vi "Configure HSDIO.vi"(8 "error in (no error)":errorcluster, 11 "HDSIO_Settings":T3={"HSDIO VISA"="6556_0", "Waveform Directory"=path "C:/Users/user/Documents/AD2240/Waveforms/RFFE6", "logic family "=8, "Clock Rate"=20000000.0, "channel list (Clock,Data)"="2,0,6"} {"Clock Rate" format="%.2p"; "logic family" items=["5.0V Logic"=5, "3.3V Logic"=6, "2.5V Logic"=7, "1.8V Logic"=8, "1.5V Logic"=80, "1.2V Logic"=81]}) -> (0 "error out":errorcluster, 3 "HSDIO Sessions":T1)   [LabVIEW 2013]
uses:
  <instrlib>/niHSDIO/niHSDIO.llb/niHSDIO_ctl Voltage Logic Family Values (Ring).ctl
  <instrlib>/niHSDIO/niHSDIO.llb/niHSDIO_ctl Trigger Script - trigID Values (Ring).ctl
  <instrlib>/niHSDIO/niHSDIO.llb/niHSDIO_ctl Generation Mode Values (Ring).ctl
  <instrlib>/niHSDIO/niHSDIO.llb/niHSDIO_ctl Data Position Values (Ring).ctl
  <instrlib>/niHSDIO/niHSDIO.llb/niHSDIO_ctl Trigger Source Values (Ring).ctl
  <instrlib>/niHSDIO/niHSDIO.llb/niHSDIO_ctl Exported Signal Name Values (Ring).ctl
  <instrlib>/niHSDIO/niHSDIO.llb/niHSDIO Configure Data Voltage Logic Family.vi
  <instrlib>/niHSDIO/niHSDIO.llb/niHSDIO Configure Initial State (String).vi
  <instrlib>/niHSDIO/niHSDIO.llb/niHSDIO Configure Idle State (String).vi
  <instrlib>/niHSDIO/niHSDIO.llb/niHSDIO Configure Software Script Trigger.vi
  <instrlib>/niHSDIO/niHSDIO.llb/niHSDIO Configure Digital Edge Start Trigger.vi
  <instrlib>/niHSDIO/niHSDIO.llb/niHSDIO Write Named Waveform From File (HWS).vi
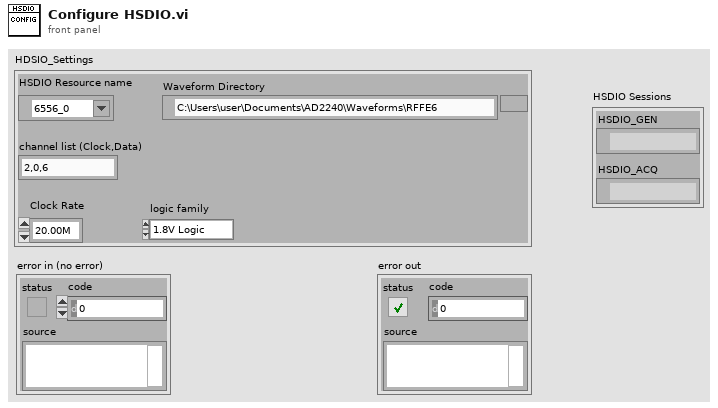
[diagram p1: front panel]
types:
  T1 = cluster{"HSDIO_ACQ":refnum<k15>, "HSDIO_GEN":refnum<k15>}
  T2 = typedef "niHSDIO_ctl Voltage Logic Family Values (Ring).ctl" = i32
  T3 = cluster{"HSDIO VISA":refnum<k15>, "Waveform Directory":path, "logic family ":T2, "Clock Rate":dbl, "channel list (Clock,Data)":string}
  T4 = typedef "niHSDIO_ctl Exported Signal Name Values (Ring).ctl" = u16
  T5 = typedef "niHSDIO_ctl Trigger Source Values (Ring).ctl" = string
  T6 = typedef "niHSDIO_ctl Data Position Values (Ring).ctl" = i32
  T7 = typedef "niHSDIO_ctl Generation Mode Values (Ring).ctl" = i32
  T8 = typedef "niHSDIO_ctl Trigger Script - trigID Values (Ring).ctl" = string
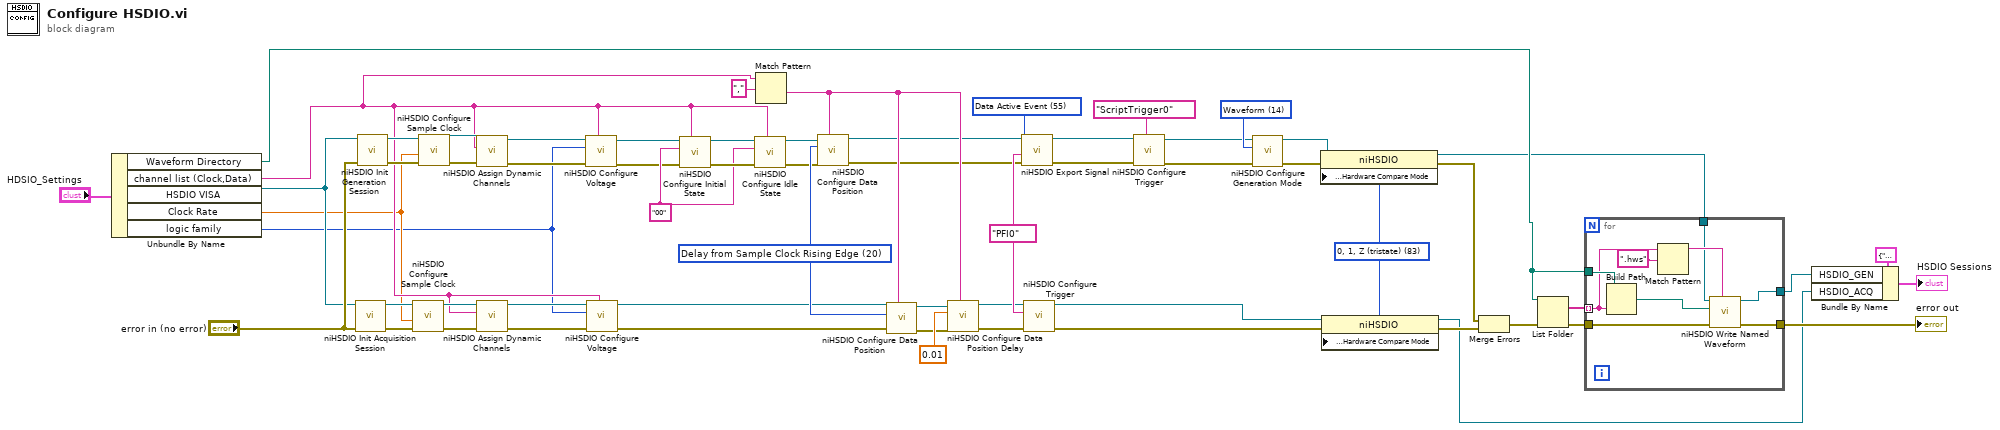
[diagram p0: block diagram]
diagram:
  w41 = "00" ("initial state")
  w49 = T4 55 items=["Sample Clock"=51, "Reference Clock"=52, "Start Trigger"=53, "Reference Trigger"=54, "Advance Trigger"=61, "Pause Trigger"=57, "Script Trigger"=58, "Stop Trigger"=82, "Data Active Event"=55, "Marker Event"=59, "Ready For Start Event"=56, "Ready For Advance Event"=66, "End Of Record Event"=68, "Onboard Ref Clock"=60] ("signal (sample clock)")
  w48 = T5 "PFI0" ("source (PFI 0)")
  w54 = 83 items=["0, 1 (binary)"=77, "0, 1, Z (tristate)"=83, "0, 1, Z, L, H, X (stim/resp)"=78, "L, H, X (resp only)"=79] ("Advanced:Supported Data States")
  w53 = T6 20 items=["Sample Clock Rising Edge"=18, "Sample Clock Falling Edge"=19, "Delay from Sample Clock Rising Edge"=20] ("position (rising edge)")
  w57 = T7 14 items=["Waveform"=14, "Scripted"=15] ("generation mode (waveform)")
  n1 = Unbundle By Name("HDSIO_Settings") -> ("Waveform Directory"=w6:path, "channel list (Clock,Data)"=w9:string, "HSDIO VISA"=w10:refnum<k15>, "Clock Rate"=w8:dbl, "logic family"=w7:T2)
  n2 = call <instrlib>:"niHSDIO Init Acquisition Session.vi"("error in (no error)"="error in (no error)", "resource name"=w10) -> ("error out"=w40:errorcluster, "instrument handle out"=w44:refnum<k15>)  [unwired: 8 in]
  n3 = call <instrlib>:"niHSDIO Init Generation Session.vi"("error in (no error)"="error in (no error)", "resource name"=w10) -> ("error out"=w43:errorcluster, "instrument handle out"=w45:refnum<k15>)  [unwired: 8 in]
  n4 = call <instrlib>:"niHSDIO Configure Sample Clock.vi"("error in (no error)"=w40, "clock rate (50MHz)"=w8, "instrument handle"=w44) -> ("error out"=w56:errorcluster, "instrument handle out"=w55:refnum<k15>)  [unwired: 7 in]
  n5 = call <instrlib>:"niHSDIO Configure Sample Clock.vi"("error in (no error)"=w43, "clock rate (50MHz)"=w8, "instrument handle"=w45) -> ("error out"=w60:errorcluster, "instrument handle out"=w59:refnum<k15>)  [unwired: 7 in]
  n6 = call <instrlib>:"niHSDIO Assign Dynamic Channels.vi"("error in (no error)"=w60, "channel list (all:\"\")"=w9, "instrument handle"=w59) -> ("error out"=w37:errorcluster, "instrument handle out"=w36:refnum<k15>)  [unwired: 7 in]
  n7 = call <instrlib>:"niHSDIO Assign Dynamic Channels.vi"("error in (no error)"=w56, "channel list (all:\"\")"=w9, "instrument handle"=w55) -> ("error out"=w35:errorcluster, "instrument handle out"=w34:refnum<k15>)  [unwired: 7 in]
  n8 = call-poly <instrlib>:"niHSDIO Configure Voltage.vi"("channel list (all:\"\")"=w9, "error in (no error)"=w37, "logic family (3.3V logic)"=w7, "instrument handle"=w36) -> ("error out"=w33:errorcluster, "instrument handle out"=w32:refnum<k15>)  [unwired: 6 in]
  n9 = call-poly <instrlib>:"niHSDIO Configure Voltage.vi"("channel list (all:\"\")"=w9, "error in (no error)"=w35, "logic family (3.3V logic)"=w7, "instrument handle"=w34) -> ("error out"=w29:errorcluster, "instrument handle out"=w28:refnum<k15>)  [unwired: 6 in]
  n10 = call-poly <instrlib>:"niHSDIO Configure Initial State.vi"("channel list"=w9, "error in (no error)"=w33, "initial state"=w41, "instrument handle"=w32) -> ("error out"=w47:errorcluster, "instrument handle out"=w46:refnum<k15>)  [unwired: 6 in]
  n11 = call-poly <instrlib>:"niHSDIO Configure Idle State.vi"("channel list"=w9, "error in (no error)"=w47, "idle state"=w41, "instrument handle"=w46) -> ("error out"=w31:errorcluster, "instrument handle out"=w30:refnum<k15>)  [unwired: 6 in]
  n12 = Match Pattern(string=w9, regular expression=",") -> (after substring=w38:string)  [unwired: 1 in, 3 out]
  n13 = call <instrlib>:"niHSDIO Configure Data Position.vi"("channel list (all:\"\")"=w38, "error in (no error)"=w31, "position (rising edge)"=w53, "instrument handle"=w30) -> ("error out"=w27:errorcluster, "instrument handle out"=w26:refnum<k15>)  [unwired: 6 in]
  n14 = call <instrlib>:"niHSDIO Configure Data Position.vi"("channel list (all:\"\")"=w38, "error in (no error)"=w29, "position (rising edge)"=w53, "instrument handle"=w28) -> ("error out"=w50:errorcluster, "instrument handle out"=w51:refnum<k15>)  [unwired: 6 in]
  n15 = call <instrlib>:"niHSDIO Configure Data Position Delay.vi"("channel list (all:\"\")"=w38, "error in (no error)"=w50, "delay (0.000)"=0.01, "instrument handle"=w51) -> ("error out"=w25:errorcluster, "instrument handle out"=w24:refnum<k15>)  [unwired: 6 in]
  n16 = call <instrlib>:"niHSDIO Export Signal.vi"("error in (no error)"=w27, "output terminal (do not export)"=w48, "signal (sample clock)"=w49, "instrument handle"=w26) -> ("error out"=w23:errorcluster, "instrument handle out"=w22:refnum<k15>)  [unwired: 6 in]
  n17 = call-poly <instrlib>:"niHSDIO Configure Trigger.vi"("error in (no error)"=w25, "source (PFI 0)"=w48, "instrument handle"=w24) -> ("error out"=w19:errorcluster, "instrument handle out"=w18:refnum<k15>)  [unwired: 7 in]
  n18 = call-poly <instrlib>:"niHSDIO Configure Trigger.vi"("trigger id (script trigger 0)"=T8 "ScriptTrigger0", "error in (no error)"=w23, "instrument handle"=w22) -> ("error out"=w21:errorcluster, "instrument handle out"=w20:refnum<k15>)  [unwired: 7 in]
  n19 = call <instrlib>:"niHSDIO Configure Generation Mode.vi"("error in (no error)"=w21, "generation mode (waveform)"=w57, "instrument handle"=w20) -> ("error out"=w17:errorcluster, "instrument handle out"=w16:refnum<k15>)  [unwired: 7 in]
  n20 = property on="Property Node" class="niHSDIO"(reference=w16, error in=w17, "Advanced:Hardware Compare:Hardware Compare Mode"=w54) -> (reference out=w5:refnum<k15>, error out=w14:errorcluster)
  n21 = property on="Property Node" class="niHSDIO"(reference=w18, error in=w19, "Advanced:Hardware Compare:Hardware Compare Mode"=w54) -> (reference out=w2:refnum<k15>, error out=w15:errorcluster)
  n22 = Merge Errors(w14, w15) -> (w13:errorcluster)
  n23 = List Folder(path=w6, error in=w13) -> (filenames=w61:string[], error out=w62:errorcluster)  [unwired: 2 in, 2 out]
  n24 = for {
    tunnel: [w71] -> w12
    tunnel: [w70] -> w3
    tunnel: w61 -> [w66] mode=indexing
    tunnel: w6 -> [w68]
    tunnel: w62 -> [w69]
    tunnel: w5 -> [w63]
    n25 = Build Path(base path=w68, name or relative path=w66) -> (appended path=w67:path)
    n26 = Match Pattern(string=w66, regular expression=".hws") -> (before substring=w64:string)  [unwired: 1 in, 3 out]
    n27 = call-poly <instrlib>:"niHSDIO Write Named Waveform.vi"("waveform name (default:\"\")"=w64, "error in (no error)"=w69, "file path"=w67, "instrument handle"=w63) -> ("error out"=w71:errorcluster, "instrument handle out"=w70:refnum<k15>)  [unwired: 5 in, 1 out]
  }
  "error out" <- w12
  n28 = Bundle By Name(cluster=T1 {"HSDIO_ACQ"="", "HSDIO_GEN"=""} ("HSDIO Sessions"), "HSDIO_GEN"=w3, "HSDIO_ACQ"=w2) -> (→"HSDIO Sessions":T1)
